vi "Handle Collapse Event.vi"(8 "error in (no error)":errorcluster, 10 "Collapse?":bool, 11 "GVIWebProcessorApp in":refnum<class "GVIWebProcessorApp.lvclass">) -> (0 "error out":errorcluster, 3 "GVIWebProcessorApp out":refnum<class "GVIWebProcessorApp.lvclass">)   [LabVIEW 2020, in "PicoG-Processor.lvlib" / "GVIWebProcessorApp.lvclass"]
uses:
  GVIWebProcessorApp.lvclass
  Collapse Animation Done Callback.vi
  Expanding Animation Done Callback.vi
  PicoG-Processor.lvlib
  <vilib>/IlluminatedG/IG OOPanel/OOPanel/ArrayManager/ArrayManager.lvclass
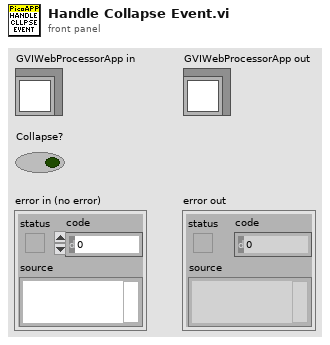
[diagram p1: front panel]
types:
  T1 = typedef "LVRectTypeDef.ctl" = cluster{"Left":i16, "Top":i16, "Right":i16, "Bottom":i16}
  T2 = typedef "PicoG-Processor.lvlib/GVIWebProcessorApp.lvclass/UI Refs.ctl" = cluster{"Main Window":refnum<vi>, "List Panel":refnum<vi>, "H Splitter":refnum<vi>, "V Splitter":refnum<vi>, "Open Project":refnum<vi>, "Project Name":refnum<vi>, "Auto Process":refnum<vi>, "Auto Deploy":refnum<vi>, "Process Platform":refnum<vi>, "Last Target":refnum<vi>}
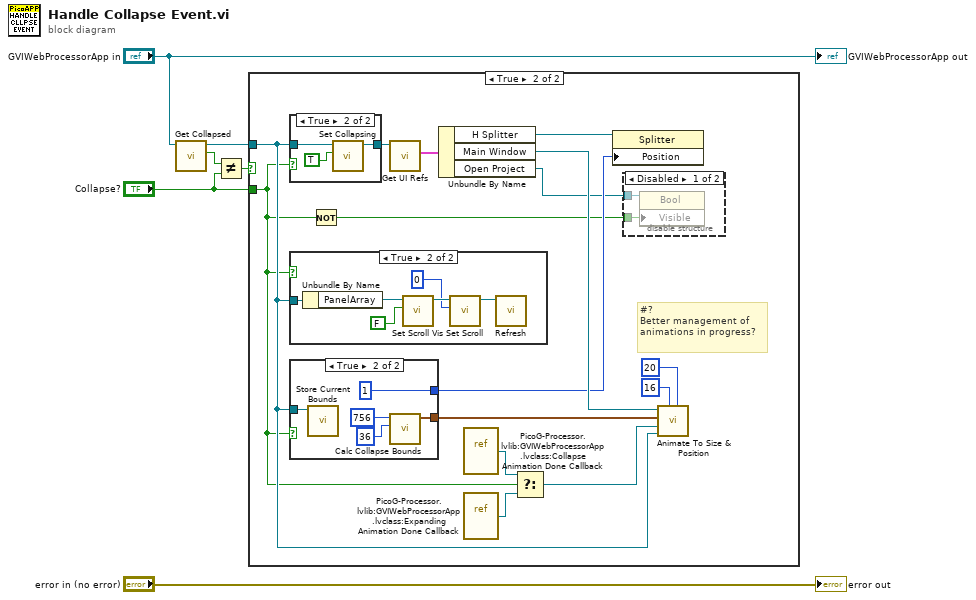
[diagram p0: block diagram]
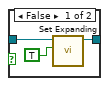
[diagram p5: hidden frame]
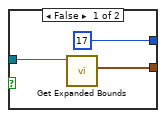
[diagram p6: hidden frame]
diagram:
  n1 = call "Get Collapsed.vi"("GVIWebProcessorApp in"="GVIWebProcessorApp in") -> ("Collapsed"=w5:bool, "GVIWebProcessorApp out"=w3:refnum<class "GVIWebProcessorApp.lvclass">)  [unwired: 8 in, 1 out]
  n2 = Not Equal?(x=w5, y="Collapse?") -> (x != y?=w4:bool)
  n3 = case shown="True" w4 {
    tunnel: "Collapse?" -> [_ w9]
    tunnel: w3 -> [_ w11]
    frame False {
      # "Already in desired state, ignore"
    }
    frame True {
      # "#?\nBetter management of animations in progress?"
      n4 = case shown="True" w9 {
        tunnel: w11 -> [w32 w34]
        tunnel: [w31 w35] -> w15
        frame False {
          n5 = call "Set Expanding.vi"("Expanding"=TRUE, "GVIWebProcessorApp in"=w32) -> ("GVIWebProcessorApp out"=w31:refnum<class "GVIWebProcessorApp.lvclass">)  [unwired: 8 in, 1 out]
        }
        frame True {
          n6 = call "Set Collapsing.vi"("Collapsing"=TRUE, "GVIWebProcessorApp in"=w34) -> ("GVIWebProcessorApp out"=w35:refnum<class "GVIWebProcessorApp.lvclass">)  [unwired: 8 in, 1 out]
        }
      }
      n7 = case shown="True" w9 {
        tunnel: w11 -> [_ w25]
        frame False {
          # "PanelArray expanding update handled in expanding animation done callback."
        }
        frame True {
          n8 = Unbundle By Name(w25) -> ("PanelArray"=w29:refnum<class "ArrayManager.lvclass">)
          n9 = call <vilib>:"Set Scroll Vis.vi"("Scroll Visible"=FALSE, "ArrayManager in"=w29) -> ("ArrayManager out"=w28:refnum<class "ArrayManager.lvclass">)  [unwired: 8 in, 1 out]
          n10 = call <vilib>:"Set Scroll.vi"("Position"=0, "ArrayManager in"=w28) -> ("ArrayManager out"=w26:refnum<class "ArrayManager.lvclass">)  [unwired: 8 in, 1 out]
          n11 = call <vilib>:"Refresh.vi"("ArrayManager in"=w26) -> ()  [unwired: 9 in, 2 out]
        }
      }
      n12 = case shown="True" w9 {
        tunnel: [w37 w41] -> w19
        tunnel: [17 ("Splitter Position") 1 ("Splitter Position")] -> w16
        tunnel: w11 -> [w36 w39]
        frame False {
          n13 = call "Get Expanded Bounds.vi"("GVIWebProcessorApp in"=w36) -> ("Expanded Bounds"=w37:T1)  [unwired: 8 in, 2 out]
        }
        frame True {
          n14 = call "Store Current Bounds.vi"("GVIWebProcessorApp in"=w39) -> ()  [unwired: 9 in, 2 out]
          n15 = call "Calc Collapse Bounds.vi"("Panel Height"=i16 36 ("Panel Width"), "Panel Width"=i16 756) -> ("Collapsed Bounds"=w41:T1)  [unwired: 9 in]
        }
      }
      n16 = Not(x=w9) -> (.not. x?=w8:bool)
      n17 = call "Get UI Refs.vi"("GVIWebProcessorApp in"=w15) -> ("UI Refs"=w10:T2)  [unwired: 8 in, 2 out]
      n18 = Unbundle By Name(w10) -> ("H Splitter"=w17:refnum<vi>, "Main Window"=w18:refnum<vi>, "Open Project"=w7:refnum<vi>)
      n19 = vi-ref "PicoG-Processor.lvlib:GVIWebProcessorApp.lvclass:Collapse Animation Done Callback.vi"() -> (w14:refnum<vi>)
      n20 = vi-ref "PicoG-Processor.lvlib:GVIWebProcessorApp.lvclass:Expanding Animation Done Callback.vi"() -> (w12:refnum<vi>)
      n21 = Select(t=w14, s=w9, f=w12) -> (s? t:f=w13:refnum<vi>)
      n22 = property class="Splitter"(reference=w17, "Position"=w16) -> ()  [unwired: 1 in, 2 out]
      n23 = disable-structure shown="Disabled" {
        disable-tunnel: w8 -> [w23 _]
        disable-tunnel: w7 -> [w22 _]
        frame Disabled {
          n24 = property class="Bool"(reference=w22, "Visible"=w23) -> ()  [unwired: 1 in, 2 out]
        }
        frame Enabled {
        }
      }
      n25 = call "Animate To Size & Position.vi"("Delay mS"=u32 20, "Steps"=16, "Callback Owner"=w11, "Done Callback"=w13, "Dest Bounds"=w19, "VI Refnum"=w18) -> ()  [unwired: 6 in]
    }
  }
  "error out" <- "error in (no error)"
  "GVIWebProcessorApp out" <- "GVIWebProcessorApp in"
